vi "Write.vi"(8 "error in (no error)":errorcluster, 10 "Statement":T1={"timestamp"=timestamp(0 s since 1904-01-01), "level"=enum."INFO", "sourceTag"="", "originVI"="", "message"=""}, 11 "ConsoleAppender in":refnum<class "ConsoleAppender.lvclass">) -> (0 "error out":errorcluster, 3 "ConsoleAppender out":refnum<class "ConsoleAppender.lvclass">)   [LabVIEW 2026, in "Lumberjack.lvlib" / "ConsoleAppender.lvclass"]
doc: "Format the Statement via the held layout and print the line to the console/standard output. Override of the abstract Write (SRS-LMBR-018)."
uses:
  ConsoleAppender.lvclass
  TypeDefs/Statement.ctl
  TypeDefs/Severity.ctl
  ConsoleAppender.lvclass/ConsoleAppender.ctl
  Layouts/Layout.lvclass/Layout.lvclass
  msvcrt.dll
  Lumberjack.lvlib
panel:
  out "Bytes Written":i32
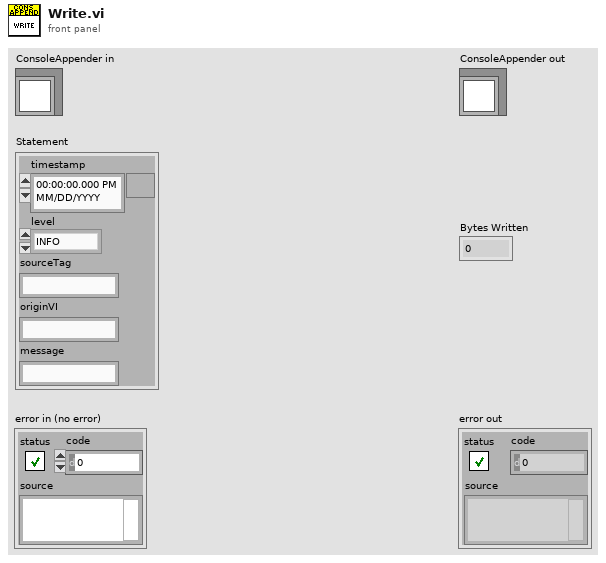
[diagram p1: front panel]
types:
  T1 = typedef "Lumberjack.lvlib/Statement.ctl" = cluster{"timestamp":timestamp, "level":T2, "sourceTag":string, "originVI":string, "message":string}
  T2 = typedef "Lumberjack.lvlib/Severity.ctl" = enum16{"OFF", "FATAL", "ERROR", "WARN", "INFO", "DEBUG", "TRACE", "ALL"}
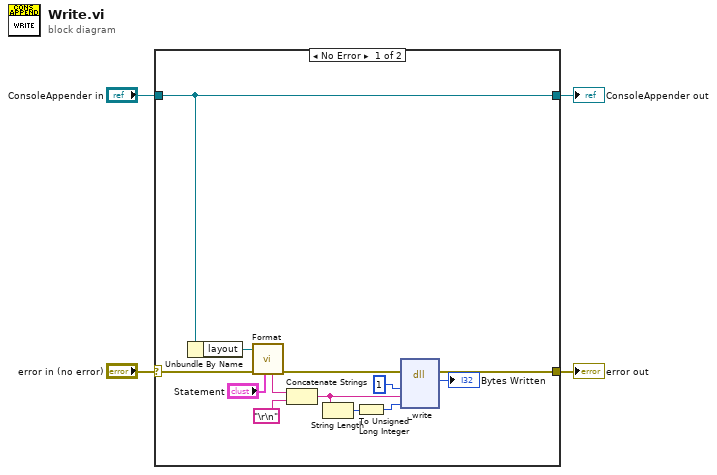
[diagram p0: block diagram]
diagram:
  n1 = case shown="No Error" "error in (no error)" {
    selector: "error in (no error)" -> [w15 w19]
    tunnel: "ConsoleAppender in" -> [w14 w18]
    tunnel: [w12 w19] -> w3
    tunnel: [w14 w18] -> w1
    frame No Error {
      n2 = Unbundle By Name(w14) -> ("layout"=w17:refnum<class "Layout.lvclass">)
      n3 = call-dynamic "Format.vi"("Statement"="Statement", "error in (no error)"=w15, "Layout in"=w17) -> ("error out"=w13:errorcluster, "FormattedLine"=w11:string)  [unwired: 6 in, 1 out]
      n4 = Concatenate Strings(w11, "\r\n") -> (w8:string)
      n5 = String Length(string=w8) -> (length=w7:i32)
      n6 = To Unsigned Long Integer(number=w7) -> (unsigned 32bit integer=w6:u32)
      n7 = dll-call lib="msvcrt.dll" fn="_write"(error in=w13, "fd"=1, "buffer"=w8, "count"=w6) -> (error out=w12:errorcluster, "return type"=→"Bytes Written":i32)  [unwired: 5 in, 1 out]
    }
    frame Error {
    }
  }
  "error out" <- w3
  "ConsoleAppender out" <- w1
